vi "Format Bus Raw Log.vi"(8 "error in (no error)":errorcluster, 10 "Bus Raw Log":u16[](array[numeric]), 11 "Bus Monitor in":refnum<class "Bus Monitor.lvclass">) -> (0 "error out":errorcluster, 2 "Formatted Log":string[][](array[string]), 3 "Bus Monitor out":refnum<class "Bus Monitor.lvclass">)   [LabVIEW 2016, in "BCI-1553 API.lvlib" / "Bus Monitor.lvclass"]
doc: "Converts a raw bus monitor log to a human-readable format. The first row is a header."
uses:
  Bus Monitor.lvclass
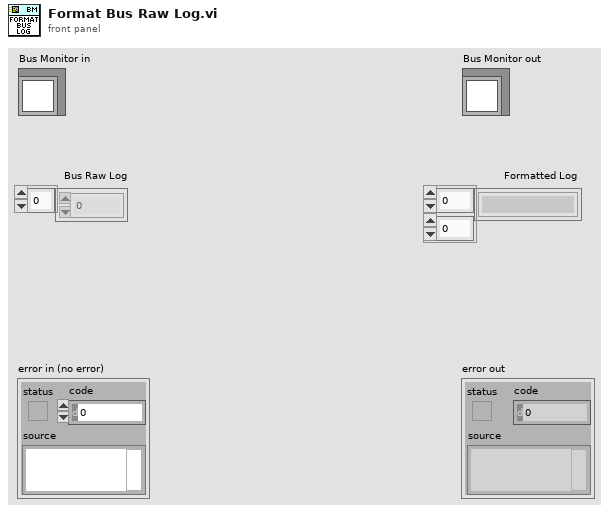
[diagram p1: front panel]
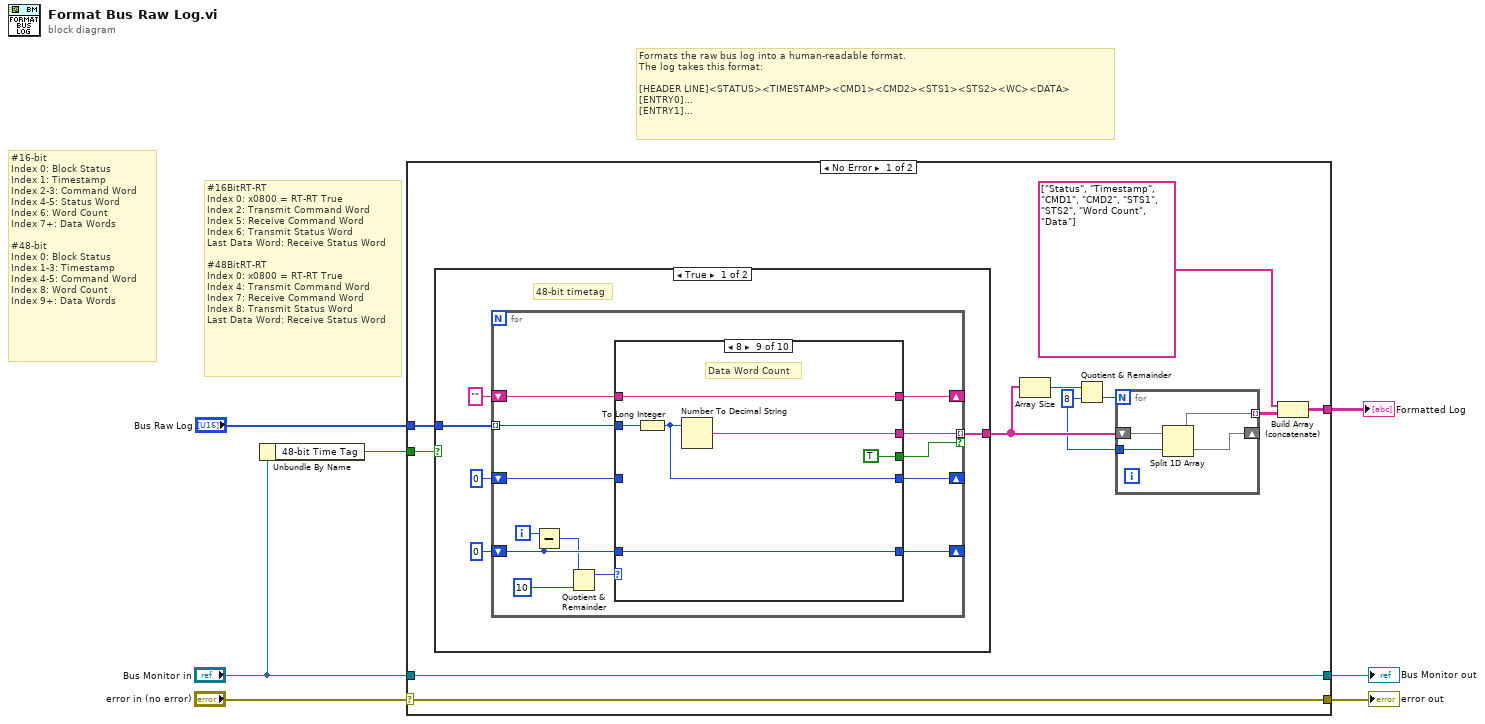
[diagram p0: block diagram]
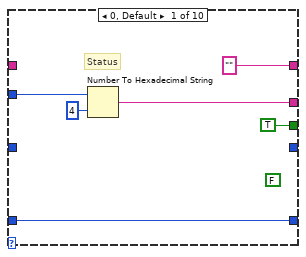
[diagram p2: hidden frame]
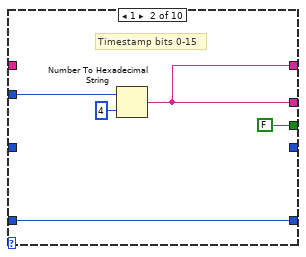
[diagram p3: hidden frame]
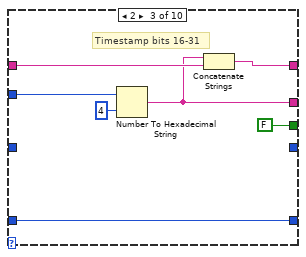
[diagram p4: hidden frame]
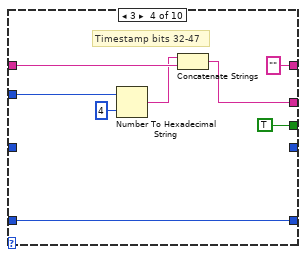
[diagram p5: hidden frame]
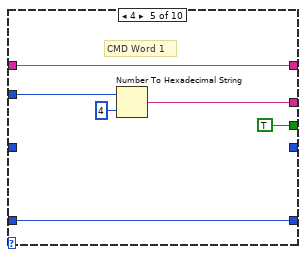
[diagram p6: hidden frame]
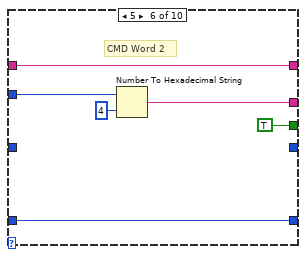
[diagram p7: hidden frame]
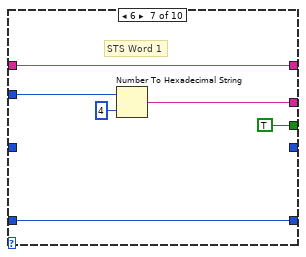
[diagram p8: hidden frame]
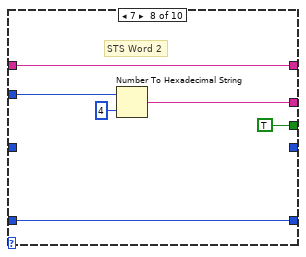
[diagram p9: hidden frame]
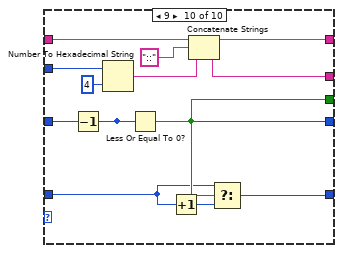
[diagram p10: hidden frame]
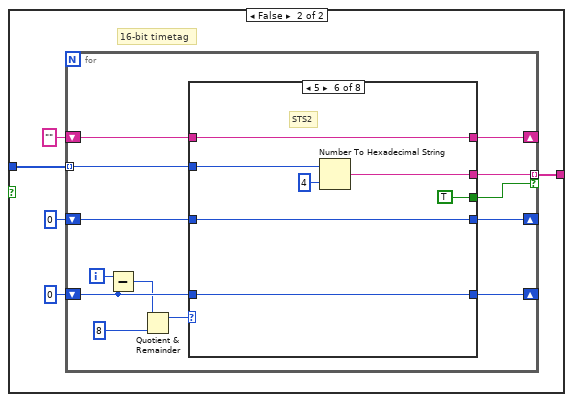
[diagram p11: hidden frame]
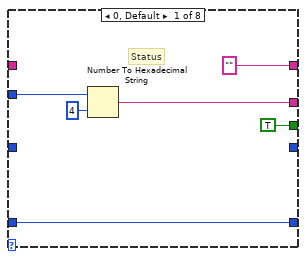
[diagram p12: hidden frame]
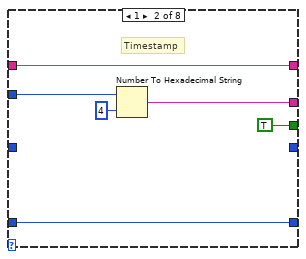
[diagram p13: hidden frame]
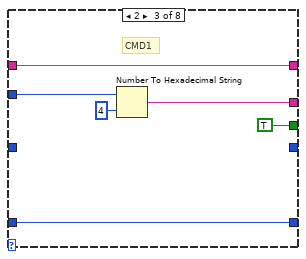
[diagram p14: hidden frame]
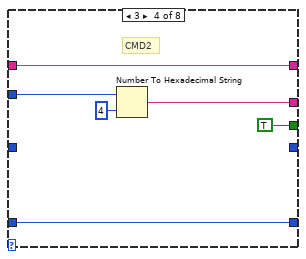
[diagram p15: hidden frame]
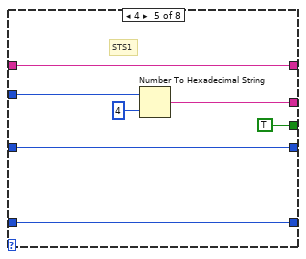
[diagram p16: hidden frame]
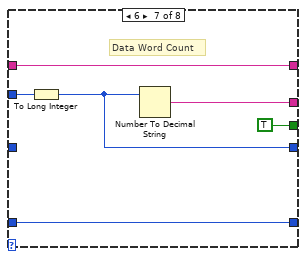
[diagram p17: hidden frame]
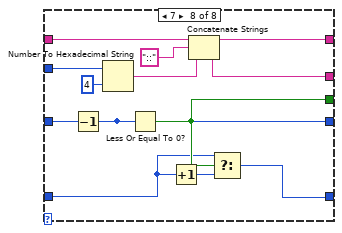
[diagram p18: hidden frame]
diagram:
  # "#16BitRT-RT\nIndex 0: x0800 = RT-RT True\nIndex 2: Transmit Command Word\nIndex 5: Receive Command Word\nIndex 6: Transmit Status Word\nLast Data Word: Receive Status Word\n\n#48BitRT-RT\nIndex 0: x0800 = RT-RT True\nIndex 4: Transmit Command Word\nIndex 7: Receive Command Word\nIndex 8: Transmit Status Word\nLast Data Word: Receive Status Word"
  # "#16-bit\nIndex 0: Block Status\nIndex 1: Timestamp\nIndex 2-3: Command Word\nIndex 4-5: Status Word\nIndex 6: Word Count\nIndex 7+: Data Words\n\n#48-bit\nIndex 0: Block Status\nIndex 1-3: Timestamp\nIndex 4-5: Command Word\nIndex 8: Word Count\nIndex 9+: Data Words"
  # "Formats the raw bus log into a human-readable format.\nThe log takes this format:\n\n[HEADER LINE]<STATUS><TIMESTAMP><CMD1><CMD2><STS1><STS2><WC><DATA>\n[ENTRY0]...\n[ENTRY1]..."
  n1 = Unbundle By Name("Bus Monitor in") -> ("48-bit Time Tag"=w1:bool)
  n2 = case shown="No Error" "error in (no error)" {
    selector: "error in (no error)" -> [w17 w184]
    tunnel: [w17 w184] -> w6
    tunnel: [w18 w183] -> w5
    tunnel: "Bus Monitor in" -> [w18 w183]
    tunnel: "Bus Raw Log" -> [w16 _]
    tunnel: [w10 _] -> w3
    tunnel: w1 -> [w8 _]
    frame No Error {
      w12 = 8 ("y")
      n3 = case shown="True" w8 {
        tunnel: w16 -> [w23 w109]
        tunnel: [w19 w105] -> w15
        frame True {
          # "48-bit timetag"
          n4 = for {
            tunnel: w23 -> [w30] mode=indexing
            shift-right: [w34] -> _
            shift-left: 0 ("y") -> [w32]
            tunnel: [w29] -> w19 mode=indexing if=w26
            shift-right: [w28] -> _
            shift-left: "" -> [w27]
            shift-right: [w25] -> _
            shift-left: 0 -> [w24]
            i -> [w33]
            n5 = Subtract(x=w33, y=w32) -> (x-y=w31:i32)
            n6 = Quotient & Remainder(x=w31, y=10) -> (x-y*floor(x/y)=w35:i32)  [unwired: 1 out]
            n7 = case shown="8" w35 {
              tunnel: w32 -> [w42 w47 w54 w62 w68 w74 w80 w86 w88 w98]
              tunnel: [w42 w47 w54 w62 w68 w74 w80 w86 w88 w96] -> w34
              tunnel: w30 -> [w37 w45 w52 w60 w65 w71 w77 w83 w90 w104]
              tunnel: [w40 w43 w49 w55 w64 w70 w76 w82 w89 w100] -> w29
              tunnel: ["" w43 w48 "" w67 w73 w79 w85 w92 w100] -> w28
              tunnel: w27 -> [_ _ w50 w57 w67 w73 w79 w85 w92 w94]
              tunnel: [TRUE FALSE FALSE TRUE TRUE TRUE TRUE TRUE TRUE w99] -> w26
              tunnel: [_ _ _ _ _ _ _ _ w87 w95] -> w25
              tunnel: w24 -> [_ _ _ _ _ _ _ _ _ w102]
              frame 0, Default {
                (unwired) FALSE
                # "Status"
                n8 = Number To Hexadecimal String(1:i16 4 ("width (-)"), 2:w37) -> (0:w40:string)
              }
              frame 1 {
                # "Timestamp bits 0-15"
                n9 = Number To Hexadecimal String(1:i16 4 ("width (-)"), 2:w45) -> (0:w43:string)
              }
              frame 2 {
                # "Timestamp bits 16-31"
                n10 = Number To Hexadecimal String(1:i16 4 ("width (-)"), 2:w52) -> (0:w49:string)
                n11 = Concatenate Strings(w49, w50) -> (w48:string)
              }
              frame 3 {
                # "Timestamp bits 32-47"
                n12 = Number To Hexadecimal String(1:i16 4 ("width (-)"), 2:w60) -> (0:w56:string)
                n13 = Concatenate Strings(w56, w57) -> (w55:string)
              }
              frame 4 {
                # "CMD Word 1"
                n14 = Number To Hexadecimal String(1:i16 4 ("width (-)"), 2:w65) -> (0:w64:string)
              }
              frame 5 {
                # "CMD Word 2"
                n15 = Number To Hexadecimal String(1:i16 4 ("width (-)"), 2:w71) -> (0:w70:string)
              }
              frame 6 {
                # "STS Word 1"
                n16 = Number To Hexadecimal String(1:i16 4 ("width (-)"), 2:w77) -> (0:w76:string)
              }
              frame 7 {
                # "STS Word 2"
                n17 = Number To Hexadecimal String(1:i16 4 ("width (-)"), 2:w83) -> (0:w82:string)
              }
              frame 8 {
                # "Data Word Count"
                n18 = To Long Integer(number=w90) -> (32bit integer=w87:i32)
                n19 = Number To Decimal String(number=w87) -> (decimal integer string=w89:string)  [unwired: 1 in]
              }
              frame 9 {
                n20 = Decrement(x=w102) -> (x-1=w95:i32)
                n21 = Number To Hexadecimal String(1:i16 4 ("width (-)"), 2:w104) -> (0:w93:string)
                n22 = Less Or Equal To 0?(x=w95) -> (x <= 0?=w99:bool)
                n23 = Increment(x=w98) -> (x+1=w97:i32)
                n24 = Concatenate Strings(w94, "::" ("string"), w93) -> (w100:string)
                n25 = Select(t=w98, s=w99, f=w97) -> (s? t:f=w96:i32)
              }
            }
          }
        }
        frame False {
          # "16-bit timetag"
          n26 = for {
            tunnel: w109 -> [w116] mode=indexing
            shift-right: [w120] -> _
            shift-left: 0 ("y") -> [w118]
            tunnel: [w115] -> w105 mode=indexing if=w112
            shift-right: [w114] -> _
            shift-left: "" -> [w113]
            shift-right: [w111] -> _
            shift-left: 0 -> [w110]
            i -> [w119]
            n27 = Subtract(x=w119, y=w118) -> (x-y=w117:i32)
            n28 = Quotient & Remainder(x=w117, y=8) -> (x-y*floor(x/y)=w121:i32)  [unwired: 1 out]
            n29 = case shown="5" w121 {
              tunnel: w118 -> [w128 w134 w140 w146 w150 w157 w162 w172]
              tunnel: [w128 w134 w140 w146 w150 w157 w162 w170] -> w120
              tunnel: w116 -> [w127 w131 w137 w143 w149 w156 w164 w178]
              tunnel: [w125 w130 w136 w142 w151 w158 w163 w174] -> w115
              tunnel: ["" w133 w139 w145 w153 w160 w166 w174] -> w114
              tunnel: w113 -> [_ w133 w139 w145 w153 w160 w166 w168]
              tunnel: [TRUE TRUE TRUE TRUE TRUE TRUE TRUE w173] -> w112
              tunnel: [_ _ _ _ w148 w155 w161 w169] -> w111
              tunnel: w110 -> [_ _ _ _ w148 w155 _ w176]
              frame 0, Default {
                # "Status"
                n30 = Number To Hexadecimal String(1:i16 4 ("width (-)"), 2:w127) -> (0:w125:string)
              }
              frame 1 {
                # "Timestamp"
                n31 = Number To Hexadecimal String(1:i16 4 ("width (-)"), 2:w131) -> (0:w130:string)
              }
              frame 2 {
                # "CMD1"
                n32 = Number To Hexadecimal String(1:i16 4 ("width (-)"), 2:w137) -> (0:w136:string)
              }
              frame 3 {
                # "CMD2"
                n33 = Number To Hexadecimal String(1:i16 4 ("width (-)"), 2:w143) -> (0:w142:string)
              }
              frame 4 {
                # "STS1"
                n34 = Number To Hexadecimal String(1:i16 4 ("width (-)"), 2:w149) -> (0:w151:string)
              }
              frame 5 {
                # "STS2"
                n35 = Number To Hexadecimal String(1:i16 4 ("width (-)"), 2:w156) -> (0:w158:string)
              }
              frame 6 {
                # "Data Word Count"
                n36 = To Long Integer(number=w164) -> (32bit integer=w161:i32)
                n37 = Number To Decimal String(number=w161) -> (decimal integer string=w163:string)  [unwired: 1 in]
              }
              frame 7 {
                n38 = Decrement(x=w176) -> (x-1=w169:i32)
                n39 = Number To Hexadecimal String(1:i16 4 ("width (-)"), 2:w178) -> (0:w167:string)
                n40 = Less Or Equal To 0?(x=w169) -> (x <= 0?=w173:bool)
                n41 = Increment(x=w172) -> (x+1=w171:i32)
                n42 = Concatenate Strings(w168, "::" ("string"), w167) -> (w174:string)
                n43 = Select(t=w172, s=w173, f=w171) -> (s? t:f=w170:i32)
              }
            }
          }
        }
      }
      n44 = Array Size(array=w15) -> (size(s)=w14:i32)
      n45 = Quotient & Remainder(x=w14, y=w12) -> (floor(x/y)=w13:i32)  [unwired: 1 out]
      n46 = for {
        N: w13 -> [_]
        tunnel: w12 -> [w179]
        shift-right: [w181] -> _
        shift-left: w15 -> [w182]
        tunnel: [w180] -> w11 mode=indexing
        n47 = Split 1D Array(array=w182, index=w179) -> (first subarray=w180:string[], second subarray=w181:string[])
      }
      n48 = Build Array (concatenate)(string[] ["Status", "Timestamp", "CMD1", "CMD2", "STS1", "STS2", "Word Count", "Data"], w11) -> (w10:string[][])
    }
    frame Error {
    }
  }
  "error out" <- w6
  "Bus Monitor out" <- w5
  "Formatted Log" <- w3
